vi "Teleop.vi"(10 "Match Info":T2={"Autonomous Elapsed Seconds"=0.0, "TeleOp Elapsed Seconds"=0.0, "Disabled Elapsed Seconds"=0.0, "Visited Autonomous"=FALSE, "Visited TeleOp"=FALSE, "Visited Disabled"=FALSE, "Autonomous Settings"={"Autonomous Style"=enum."Independent", "VI Refnum"=refnum}}, 11 "Call Context":T3) -> ()   [LabVIEW 2016]
doc: "This VI is called for each TeleOp packet received from the DS where the robot is not disabled. It is often used to read from the joysticks and update I/O or to update setpoints for timed control loops. It should complete and return within 20 milliseconds or it may miss DS packets."
uses:
  <vilib>/Rock Robotics/WPI/DriverStation/WPI_DriverStationDerivedRobotMode.ctl
  <vilib>/Rock Robotics/WPI/DriverStation/WPI_DriverStationMatch Info.ctl
  <vilib>/Rock Robotics/WPI/ThirdParty/CanMotor/CTRLib-LV-TalonSRX/Framework/ServoParams.ctl
  <vilib>/Rock Robotics/WPI/ThirdParty/CanMotor/CTRLib-LV-TalonSRX/CTRE_CANTalonSRX_ControlMode.ctl
  <vilib>/Rock Robotics/WPI/Utilities/WPI_GetSetVariantRefNum.vi
panel:
  in  "Servo Params 2":T1
  in  "Servo Params":T1
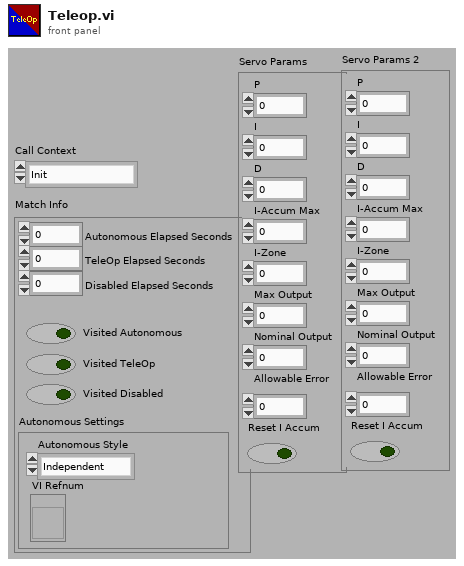
[diagram p1: front panel]
types:
  T1 = typedef "ServoParams.ctl" = cluster{"P":dbl, "I":dbl, "D":dbl, "I-Accum Max":dbl, "I-Zone":dbl, "Max Output":dbl, "Nominal Output":dbl, "Allowable Error":dbl, "Reset I Accum":bool}
  T2 = typedef "WPI_DriverStationMatch Info.ctl" = cluster{"Autonomous Elapsed Seconds":dbl, "TeleOp Elapsed Seconds":dbl, "Disabled Elapsed Seconds":dbl, "Visited Autonomous":bool, "Visited TeleOp":bool, "Visited Disabled":bool, "Autonomous Settings":cluster{"Autonomous Style":enum16{"Iterative", "Independent"}, "VI Refnum":refnum<vi>}}
  T3 = typedef "WPI_DriverStationDerivedRobotMode.ctl" = enum16{"Init", "Execute", "Stop"}
  T4 = typedef "CTRE_CANTalonSRX_ControlMode.ctl" = enum16{"Throttle (Duty-Cycle)", "Position Closed-Loop", "Velocity Closed-Loop", "Current Closed-Loop", "Voltage Compensation", "Slave Follower", "Motion Profile", "Motion Magic"}
  T5 = typedef "WPI_JoystickDevRef.ctl" = cluster{"Device":T6}
  T6 = typedef "WPI_JoystickDeviceEnum.ctl" = enum16{"USB 0", "USB 1", "USB 2", "USB 3", "USB 4", "USB 5"}
  T7 = typedef "CTRE_PigeonIMU_DeviceRef.ctl" = cluster{"DeviceStatus":errorcluster, "Device Number":u8, "Type":T8, "Device ID":u32, "Handle":u64, "UsageFrame":u32, "Library Path":path}
  T8 = typedef "CTRE_PigeonIMU_ConnectionType.ctl" = u32
  T9 = typedef "SensoredTank.ctl" = cluster{"Sensored Gearbox Left":T10, "Sensored Gearbox Right ":T10, "Wheel Radius":dbl, "Ticks Per Revolution":dbl, "Distance Between Wheels":dbl}
  T10 = typedef "SensoredGearbox.ctl" = cluster{"Smart Motor Controller":T11, "Invert":bool, "Gear Ratio":dbl}
  T11 = typedef "WPI_MotorControlDeviceRef.ctl" = cluster{"DeviceStatus":errorcluster, "Type":T12, "PWM":cluster{"PWM Channel":T13, "DeadBand":T14}, "CAN":cluster{"Device Number":u8, "SetOutput VI Ref":variant, "GetOutput VI Ref":variant, "Enable VI Ref":variant, "Disable VI Ref":variant, "Data":variant}, "Invert":bool}
  T12 = typedef "WPI_MotorControlType.ctl" = enum16{"PWM", "CAN"}
  T13 = typedef "FPGA_DIOPWMChannel.ctl" = enum8{"PWM 0", "PWM 1", "PWM 2", "PWM 3", "PWM 4", "PWM 5", "PWM 6", "PWM 7", "PWM 8", "PWM 9", "PWM MXP 0", "PWM MXP 1", "PWM MXP 2", "PWM MXP 3", "PWM MXP 4", "PWM MXP 5", "PWM MXP 6", "PWM MXP 7", "PWM MXP 8", "PWM MXP 9", "Invalid"}
  T14 = typedef "WPI_PWMDeadband.ctl" = cluster{"Name":string, "maxPositivePwm":i32, "minPositivePwm":i32, "centerPwm":i32, "maxNegativePwm":i32, "minNegativePwm":i32, "angularRange":u16}
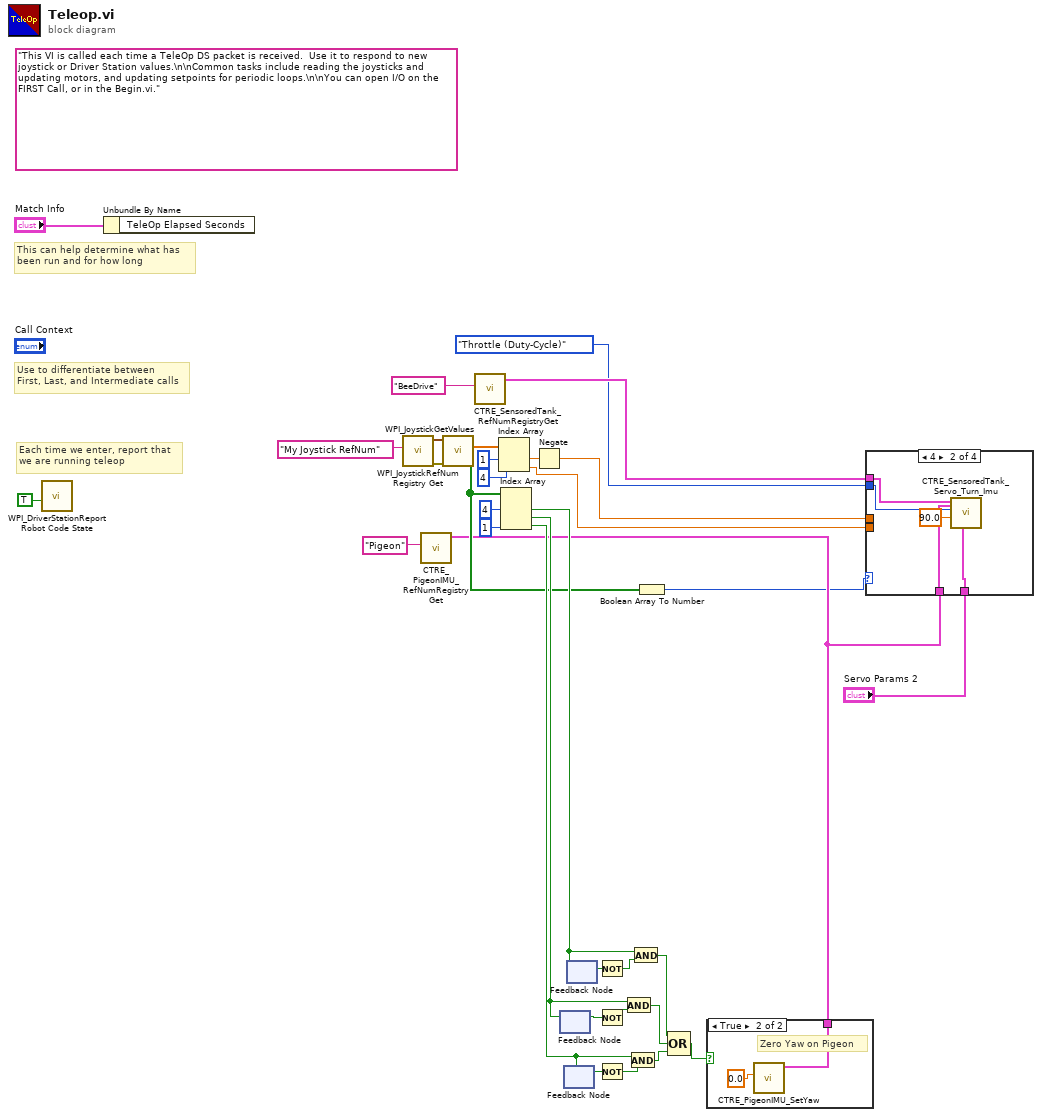
[diagram p0: block diagram]
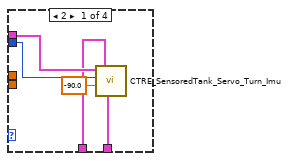
[diagram p2: hidden frame]
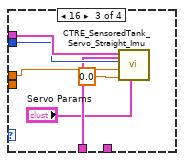
[diagram p3: hidden frame]
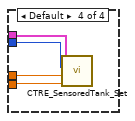
[diagram p4: hidden frame]
diagram:
  (unwired) "This VI is called each time a TeleOp DS packet is received.  Use it to respond to new joystick or Driver Station values.\n\nCommon tasks include reading the joysticks and updating motors, and updating setpoints for periodic loops.\n\nYou can open I/O on the FIRST Call, or in the Begin.vi."
  # "Each time we enter, report that\nwe are running teleop"
  # "Use to differentiate between\nFirst, Last, and Intermediate calls"
  # "This can help determine what has\nbeen run and for how long"
  n1 = call <vilib>:"WPI_DriverStationReport Robot Code State.vi"("TeleOp"=TRUE ("Autonomous")) -> ()  [unwired: 10 in, 1 out]
  n2 = Unbundle By Name("Match Info") -> ()  [unwired: 1 out]
  n3 = call <vilib>:"WPI_JoystickRefNum Registry Get.vi"("refnum name"="My Joystick RefNum") -> ("error out"=w30:errorcluster, "JoystickDevRef"=w29:T5)  [unwired: 9 in]
  n4 = call <vilib>:"CTRE_PigeonIMU_RefNumRegistryGet.vi"("refnum name"="Pigeon") -> ("PigeonIMUDevRef"=w9:T7)  [unwired: 9 in, 1 out]
  n5 = call <vilib>:"WPI_JoystickGetValues.vi"("error in (no error)"=w30, "JoystickDevRef"=w29) -> ("Buttons"=w14:bool[], "Axes"=w28:dbl[])  [unwired: 5 in, 3 out]
  n6 = call <vilib>:"CTRE_SensoredTank_RefNumRegistryGet.vi"("RefNum Name"="BeeDrive") -> ("Sensored Tank"=w13:T9)  [unwired: 10 in]
  n7 = Index Array(array=w28, index #1=1 ("index"), index #2=4 ("index")) -> (element #1=w25:dbl, element #2=w11:dbl)
  n8 = Index Array(array=w14, index #1=4 ("index"), index #2=1 ("index")) -> (element #1=w15:bool, element #2=w21:bool, element #3=w20:bool)  [unwired: 1 in]
  n9 = Negate(x=w25) -> (-x=w12:dbl)
  n10 = feedback-in #1(w21) -> ()
  n11 = feedback #1() -> (w4:bool)  [unwired: 1 in]
  n12 = feedback #2() -> (w7:bool)  [unwired: 1 in]
  n13 = feedback-in #2(w20) -> ()
  n14 = feedback #3() -> (w3:bool)  [unwired: 1 in]
  n15 = feedback-in #3(w15) -> ()
  n16 = Not(x=w3) -> (.not. x?=w2:bool)
  n17 = Not(x=w4) -> (.not. x?=w5:bool)
  n18 = Not(x=w7) -> (.not. x?=w6:bool)
  n19 = And(x=w21, y=w5) -> (x .and. y?=w19:bool)
  n20 = And(x=w20, y=w6) -> (x .and. y?=w18:bool)
  n21 = And(x=w15, y=w2) -> (x .and. y?=w16:bool)
  n22 = Boolean Array To Number(Boolean array=w14) -> (number=w8:u32)
  n23 = Compound Arithmetic op=OR(w16, w19, w18) -> (w17:bool)
  n24 = case shown="True" w17 {
    tunnel: w9 -> [_ w35]
    frame False {
    }
    frame True {
      # "Zero Yaw on Pigeon"
      n25 = call <vilib>:"CTRE_PigeonIMU_SetYaw.vi"("Value"=0.0, "PigeonIMUDevRef"=w35) -> ()  [unwired: 8 in, 2 out]
    }
  }
  n26 = case shown="4" w8 {
    tunnel: w13 -> [w40 w43 w51 w56]
    tunnel: w12 -> [_ _ w48 w55]
    tunnel: w11 -> [_ _ _ w54]
    tunnel: CTRE_CANTalonSRX_ControlMode."Throttle (Duty-Cycle)" ("Talon SRX Control Mode") -> [w38 w45 w50 w53]
    tunnel: w9 -> [w39 w44 w49 _]
    tunnel: "Servo Params 2" -> [w37 w42 _ _]
    frame 2 {
      n27 = call <vilib>:"CTRE_SensoredTank_Servo_Turn_Imu.vi"("Servo Params"=w37, "PigeonIMU"=w39, "Set Angle"=-90.0, "Talon SRX Control Mode"=w38, "Sensored Tank"=w40) -> ()  [unwired: 4 in, 3 out]
    }
    frame 4 {
      n28 = call <vilib>:"CTRE_SensoredTank_Servo_Turn_Imu.vi"("Servo Params"=w42, "PigeonIMU"=w44, "Set Angle"=90.0, "Talon SRX Control Mode"=w45, "Sensored Tank"=w43) -> ()  [unwired: 4 in, 3 out]
    }
    frame 16 {
      n29 = call <vilib>:"CTRE_SensoredTank_Servo_Straight_Imu.vi"("Servo Params"="Servo Params", "PigeonIMU"=w49, "Set Heading"=0.0, "Forward"=w48, "Talon SRX Control Mode"=w50, "Sensored Tank"=w51) -> ()  [unwired: 4 in, 2 out]
    }
    frame Default {
      n30 = call <vilib>:"CTRE_SensoredTank_Set.vi"("Turn"=w54, "Forward"=w55, "Talon SRX Control Mode"=w53, "Sensored Tank"=w56) -> ()  [unwired: 6 in, 2 out]
    }
  }
